vi "BUILD ARRAY MEMO.vi"(11 "data in":string[][](array[string])) -> (3 "ARRAY MEMO":string[][][](array[string]))   [LabVIEW 2019]
panel:
  out "size(s)":i32[](array[numeric])
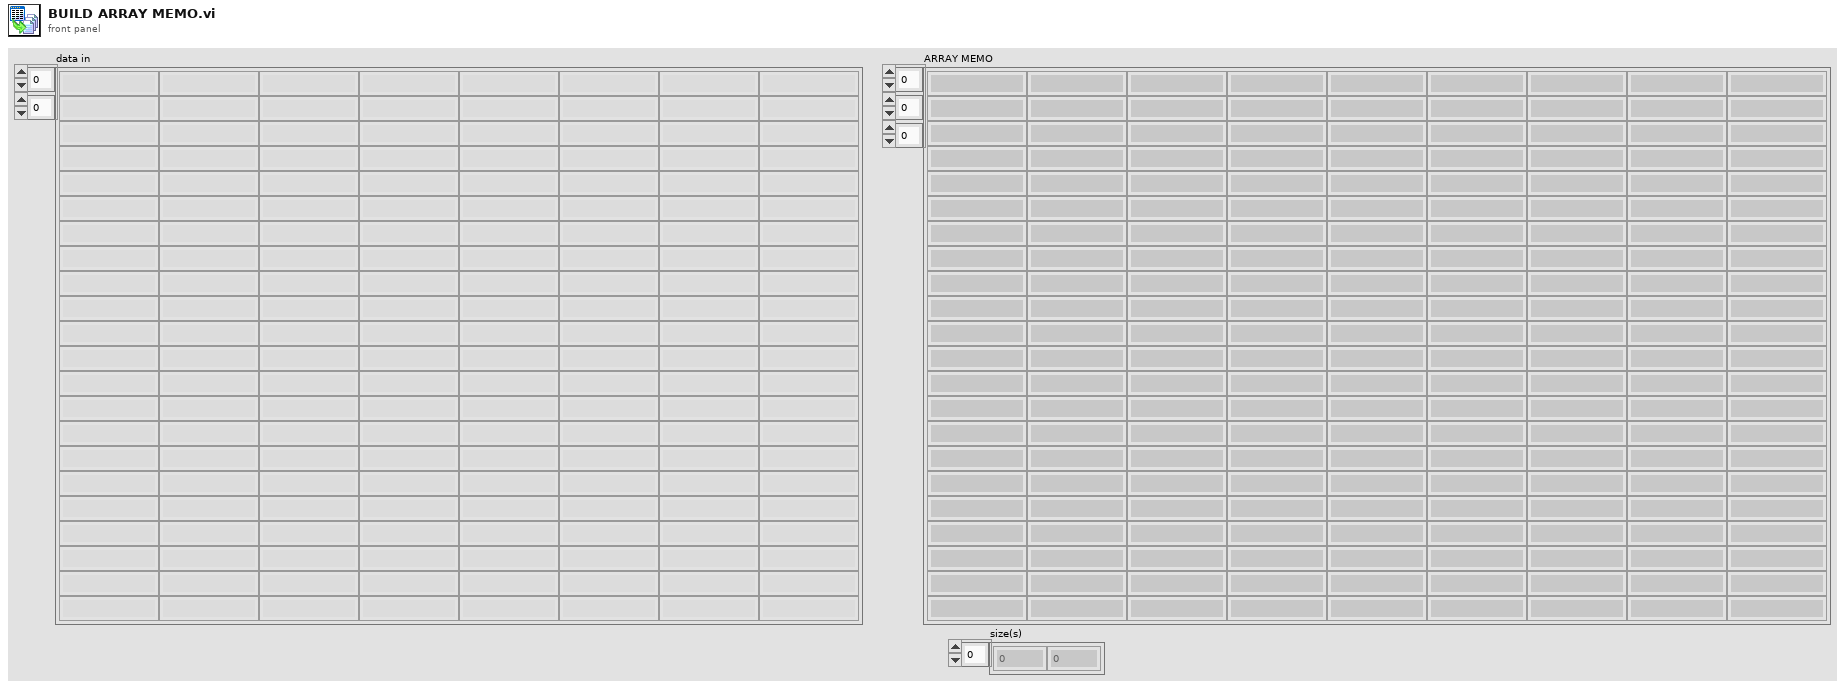
[diagram p1: front panel]
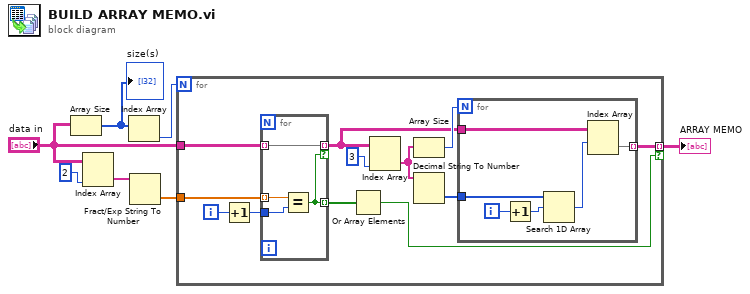
[diagram p0: block diagram]
diagram:
  n1 = Array Size(array="data in") -> (size(s)=w2:i32[])
  "size(s)" <- w2
  n2 = Index Array(array="data in", index (col)=2 ("disabled index (col)")) -> (element=w5:string[])  [unwired: 1 in]
  n3 = Index Array(array=w2) -> (element=w1:i32)  [unwired: 1 in]
  n4 = Fract/Exp String To Number(string=w5) -> (number=w7:dbl[])  [unwired: 3 in, 1 out]
  n5 = for {
    N: w1 -> [_]
    tunnel: w7 -> [w19]
    tunnel: "data in" -> [w18]
    tunnel: [w11] -> w6 mode=indexing if=w8
    i -> [w17]
    n6 = Increment(x=w17) -> (x+1=w10:i32)
    n7 = for {
      tunnel: w19 -> [w29] mode=indexing
      tunnel: w10 -> [w28]
      tunnel: w18 -> [w27] mode=indexing
      tunnel: [w27] -> w12 mode=indexing if=w26
      tunnel: [w26] -> w9 mode=indexing
      n8 = Equal?(x=w29, y=w28) -> (x = y?=w26:bool)
    }
    n9 = Or Array Elements(Boolean array=w9) -> (logical OR=w8:bool)
    n10 = Index Array(array=w12, index (col)=3 ("disabled index (col)")) -> (element=w15:string[])  [unwired: 1 in]
    n11 = Array Size(array=w15) -> (size(s)=w13:i32)
    n12 = Decimal String To Number(string=w15) -> (number=w14:i32[])  [unwired: 2 in, 1 out]
    n13 = for {
      N: w13 -> [_]
      tunnel: w14 -> [w25]
      tunnel: w12 -> [w22]
      tunnel: [w20] -> w11 mode=indexing
      i -> [w24]
      n14 = Increment(x=w24) -> (x+1=w23:i32)
      n15 = Search 1D Array(1D array=w25, element=w23) -> (index of element=w21:i32)  [unwired: 1 in]
      n16 = Index Array(array=w22, index (row)=w21) -> (element=w20:string[])  [unwired: 1 in]
    }
  }
  "ARRAY MEMO" <- w6
